vi "destroy.vi"(8 "error in (no error)":errorcluster, 11 "NotifierStopMechanism in":refnum<class "BoolNotifierStopMechanism.lvclass">) -> (0 "error out":errorcluster, 3 "NotifierStopMechanism out":refnum<class "BoolNotifierStopMechanism.lvclass">)   [LabVIEW 2023, in "TLC_Daemon.lvlib" / "BoolNotifierStopMechanism.lvclass"]
doc: "Destroy procedure\n_____________________________________\nTLC Daemon 1.0.0.2\nCopyright (c) 2026 Andrea Cadei"
uses:
  BoolNotifierStopMech/BoolNotifierStopMechanism.lvclass
  BoolNotifierStopMech/BoolNotifierStopMechanism.lvclass/BoolNotifierStopMechanism.ctl
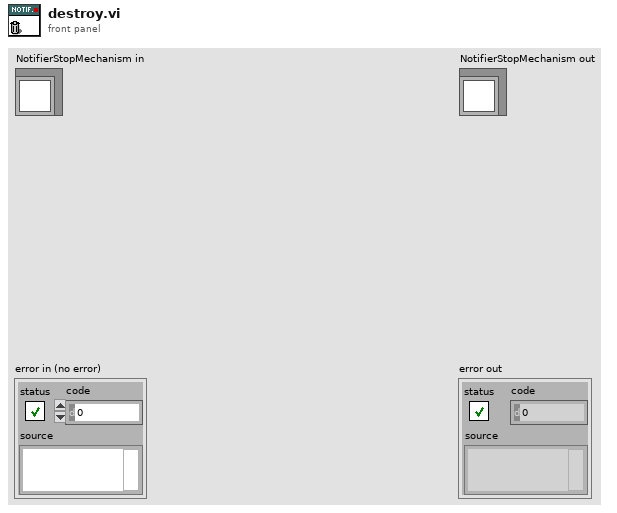
[diagram p1: front panel]
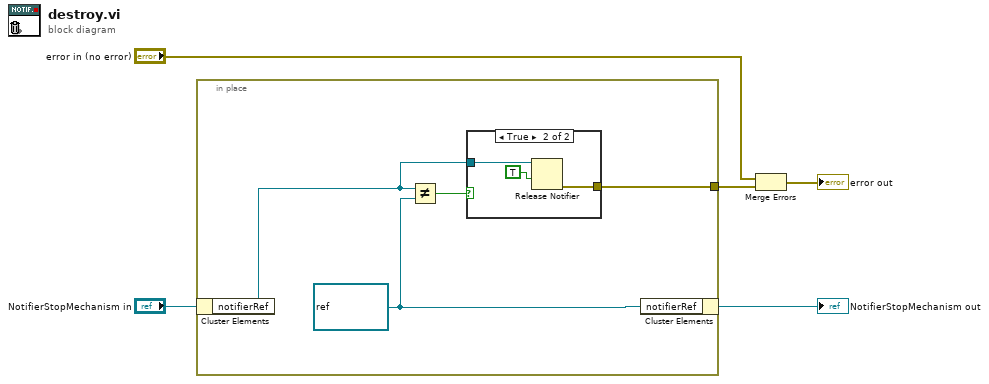
[diagram p0: block diagram]
diagram:
  n1 = in-place {
    in-place-border: [w6] -> w2
    w9 = refnum<notifier> refnum ("notifierRef")
    n2 = in-place-cluster #1("NotifierStopMechanism in") -> ("notifierRef"=w7:refnum<notifier>)
    n3 = Not Equal?(x=w7, y=w9) -> (x != y?=w8:bool)
    n4 = case shown="True" w8 {
      tunnel: w7 -> [_ w12]
      tunnel: [_ w10] -> w6
      frame False {
      }
      frame True {
        n5 = Release Notifier(notifier=w12, force destroy? (F)=TRUE) -> (error out=w10:errorcluster)  [unwired: 1 in, 2 out]
      }
    }
    n6 = in-place-cluster #1("notifierRef"=w9) -> (→"NotifierStopMechanism out":refnum<class "BoolNotifierStopMechanism.lvclass">)
  }
  n7 = Merge Errors("error in (no error)", w2) -> (→"error out":errorcluster)
